vi "雷达流速仪写调试.vi"() -> ()   [LabVIEW 2016, in "雷达流速仪.lvlib"]
panel:
  out "输出簇 5":T1
  out "输出簇 4":T1
  out "输出簇 3":T1
  out "输出簇 2":T1
  out "输出簇":T1
  in  "Error in":errorcluster caption="Error in (no error)"
  in  "雷达流速仪串口":refnum<visa-resource-name>="COM6"
  in  "波特率":u32(ring)=9600 items=["9600"=9600, "19200"=19200, "115200"=115200]
  out "error out 6":errorcluster
  out "error out 5":errorcluster
  out "error out 4":errorcluster
  out "error out 3":errorcluster
  out "error out 2":errorcluster
  out "error out 1":errorcluster
  out "数据 5":sgl
  out "数据 4":sgl
  out "数据 3":sgl
  out "数据 2":sgl
  out "数据 1":sgl
  out "采集数据":sgl[](array[numeric])
  out "error out":errorcluster
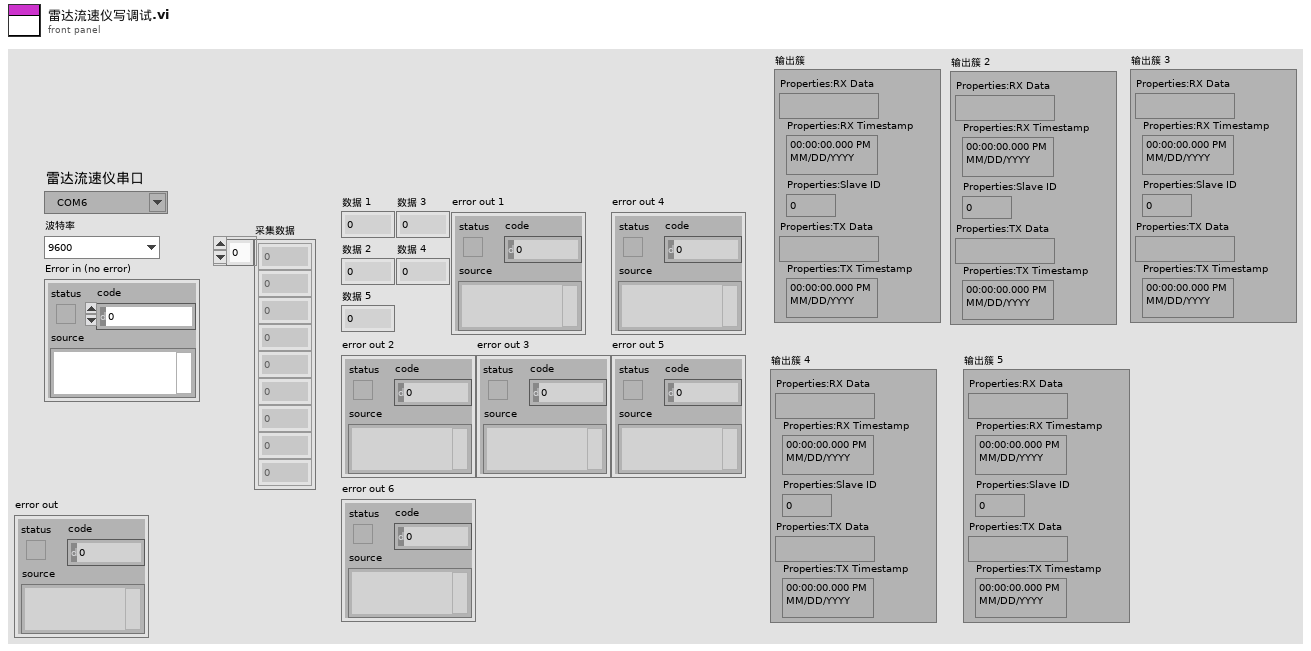
[diagram p1: front panel]
types:
  T1 = cluster{"Properties:RX Data":string, "Properties:RX Timestamp":timestamp, "Properties:Slave ID":u8, "Properties:TX Data":string, "Properties:TX Timestamp":timestamp}
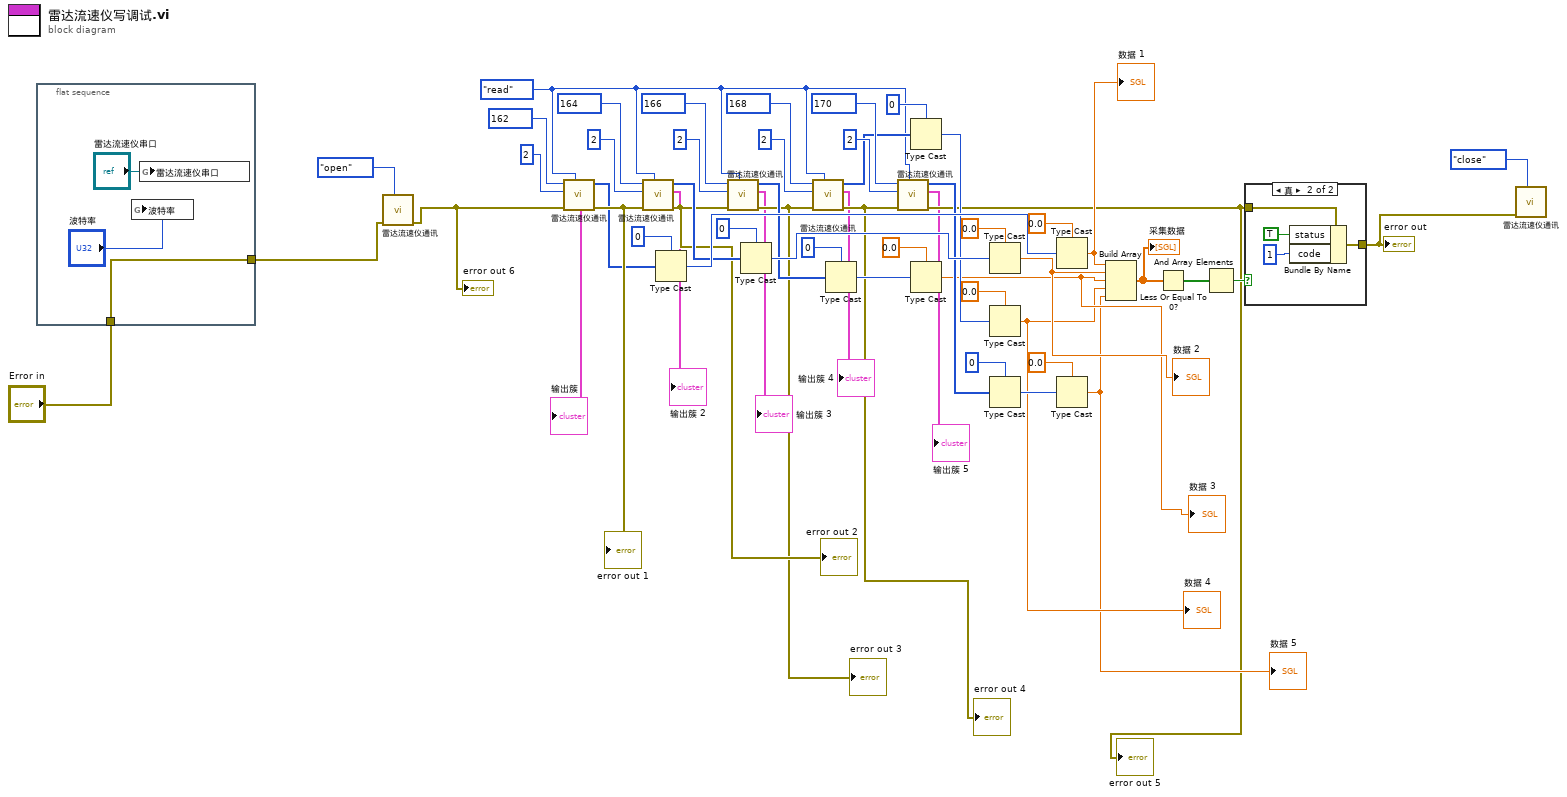
[diagram p0: block diagram]
diagram:
  w23 = enum16{"open", "read", "write", "close"}."read" ("STEP")
  n1 = flat-sequence {
    tunnel: [w56] -> w9
    tunnel: "Error in" -> [w56]
    frame #0 {
      n2 = global write "雷达流速仪全局变量.vi" "波特率"("波特率") -> ()
      n3 = global write "雷达流速仪全局变量.vi" "雷达流速仪串口"("雷达流速仪串口") -> ()
    }
  }
  n4 = call "雷达流速仪通讯.vi"("STEP"=enum16{"open", "read", "write", "close"}."open", "Error in"=w9) -> ("error out"=w10:errorcluster)  [unwired: 7 in, 2 out]
  "error out 6" <- w10
  n5 = call "雷达流速仪通讯.vi"("STEP"=w23, "Error in"=w10, "quantity"=u16 2, "starting address"=u16 162) -> ("error out"=w47:errorcluster, "输出簇"=→"输出簇":T1, "Registers"=w41:u16[])  [unwired: 5 in]
  "error out 1" <- w47
  n6 = call "雷达流速仪通讯.vi"("STEP"=w23, "Error in"=w47, "quantity"=u16 2, "starting address"=u16 164) -> ("error out"=w15:errorcluster, "输出簇"=→"输出簇 2":T1, "Registers"=w37:u16[])  [unwired: 5 in]
  "error out 2" <- w15
  n7 = Type Cast(type=u64 0, x=w41) -> (*(type *) &x=w42:u64)
  n8 = call "雷达流速仪通讯.vi"("STEP"=w23, "Error in"=w15, "quantity"=u16 2, "starting address"=u16 166) -> ("error out"=w14:errorcluster, "输出簇"=→"输出簇 3":T1, "Registers"=w33:u16[])  [unwired: 5 in]
  "error out 3" <- w14
  n9 = Type Cast(type=u64 0, x=w37) -> (*(type *) &x=w40:u64)
  n10 = call "雷达流速仪通讯.vi"("STEP"=w23, "Error in"=w14, "quantity"=u16 2, "starting address"=u16 168) -> ("error out"=w13:errorcluster, "输出簇"=→"输出簇 4":T1, "Registers"=w29:u16[])  [unwired: 5 in]
  "error out 4" <- w13
  n11 = Type Cast(type=u64 0, x=w33) -> (*(type *) &x=w34:u64)
  n12 = call "雷达流速仪通讯.vi"("STEP"=w23, "Error in"=w13, "quantity"=u16 2, "starting address"=u16 170) -> ("error out"=w12:errorcluster, "输出簇"=→"输出簇 5":T1, "Registers"=w25:u16[])  [unwired: 5 in]
  "error out 5" <- w12
  n13 = Type Cast(type=u64 0, x=w29) -> (*(type *) &x=w32:u64)
  n14 = Type Cast(type=sgl 0.0, x=w34) -> (*(type *) &x=w18:sgl)
  "数据 3" <- w18
  n15 = Type Cast(type=sgl 0.0, x=w40) -> (*(type *) &x=w19:sgl)
  "数据 2" <- w19
  n16 = Type Cast(type=sgl 0.0, x=w32) -> (*(type *) &x=w17:sgl)
  "数据 4" <- w17
  n17 = Type Cast(type=u64 0, x=w25) -> (*(type *) &x=w26:u64)
  n18 = Type Cast(type=sgl 0.0, x=w42) -> (*(type *) &x=w24:sgl)
  "数据 1" <- w24
  n19 = Type Cast(type=sgl 0.0, x=w26) -> (*(type *) &x=w16:sgl)
  "数据 5" <- w16
  n20 = Build Array(w24, w19, w18, w17, w16) -> (w22:sgl[])
  "采集数据" <- w22
  n21 = Less Or Equal To 0?(x=w22) -> (x <= 0?=w21:bool[])
  n22 = And Array Elements(Boolean array=w21) -> (logical AND=w20:bool)
  n23 = case shown="真" w20 {
    tunnel: w12 -> [w59 w63]
    tunnel: [w59 w61] -> w1
    frame False {
    }
    frame True {
      n24 = Bundle By Name(cluster=w63, "status"=TRUE, "code"=1) -> (w61:errorcluster)
    }
  }
  "error out" <- w1
  n25 = call "雷达流速仪通讯.vi"("STEP"=enum16{"open", "read", "write", "close"}."close", "Error in"=w1) -> ()  [unwired: 7 in, 3 out]
